vi "Lifschitz-Kosevich formula.vi"(3 "output control":T1, 4 "data":T2, 5 "X":dbl[](array[numeric]), 6 "a":dbl[](array[numeric])) -> (0 "error out":errorcluster, 1 "f'(X,a)":dbl[][](array[numeric]), 2 "f(X,a)":dbl[](array[numeric]))   [LabVIEW 2020]
doc: "This template is the starting point for creating a model function to be passed to the Nonlinear Curve Fit.vi."
uses:
  <vilib>/gmath/NumericalOptimization/objective function data.ctl
  <vilib>/gmath/NumericalOptimization/LM_output select.ctl
  <vilib>/gmath/NI_Gmath.lvlib
panel:
  in  "B (T)":dbl=14.69
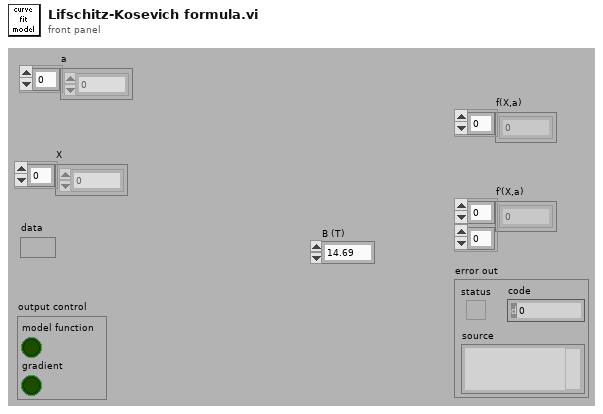
[diagram p1: front panel]
types:
  T1 = typedef "NI_Gmath.lvlib/LM_output select.ctl" = cluster{"model function":bool, "gradient":bool}
  T2 = typedef "NI_Gmath.lvlib/objective function data.ctl" = variant
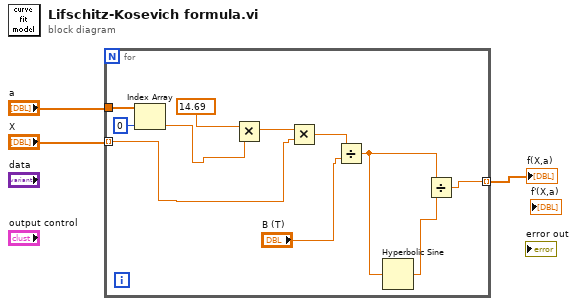
[diagram p0: block diagram]
diagram:
  n1 = for {
    tunnel: "a" -> [w7]
    tunnel: "X" -> [w8] mode=indexing
    tunnel: [w4] -> w1 mode=indexing
    n2 = Index Array(array=w7, index=0) -> (element=w5:dbl)
    n3 = Multiply(x=14.69, y=w5) -> (x*y=w13:dbl)
    n4 = Multiply(x=w13, y=w8) -> (x*y=w12:dbl)
    n5 = Divide(x=w12, y="B (T)") -> (x/y=w11:dbl)
    n6 = Hyperbolic Sine(1:w11) -> (0:w10:dbl)
    n7 = Divide(x=w11, y=w10) -> (x/y=w4:dbl)
  }
  "f(X,a)" <- w1
